vi "IR converter.vi"(1 "IR in":T1) -> (0 "distance out":T1)   [LabVIEW 2019]
uses:
  IR out.ctl
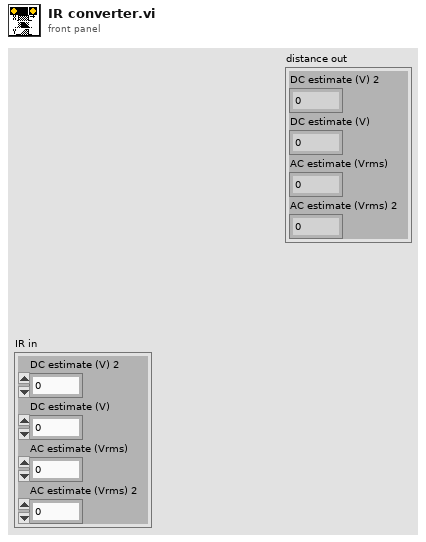
[diagram p1: front panel]
types:
  T1 = typedef "IR out.ctl" = cluster{"DC estimate (V) 2":dbl, "DC estimate (V)":dbl, "AC estimate (Vrms)":dbl, "AC estimate (Vrms) 2":dbl}
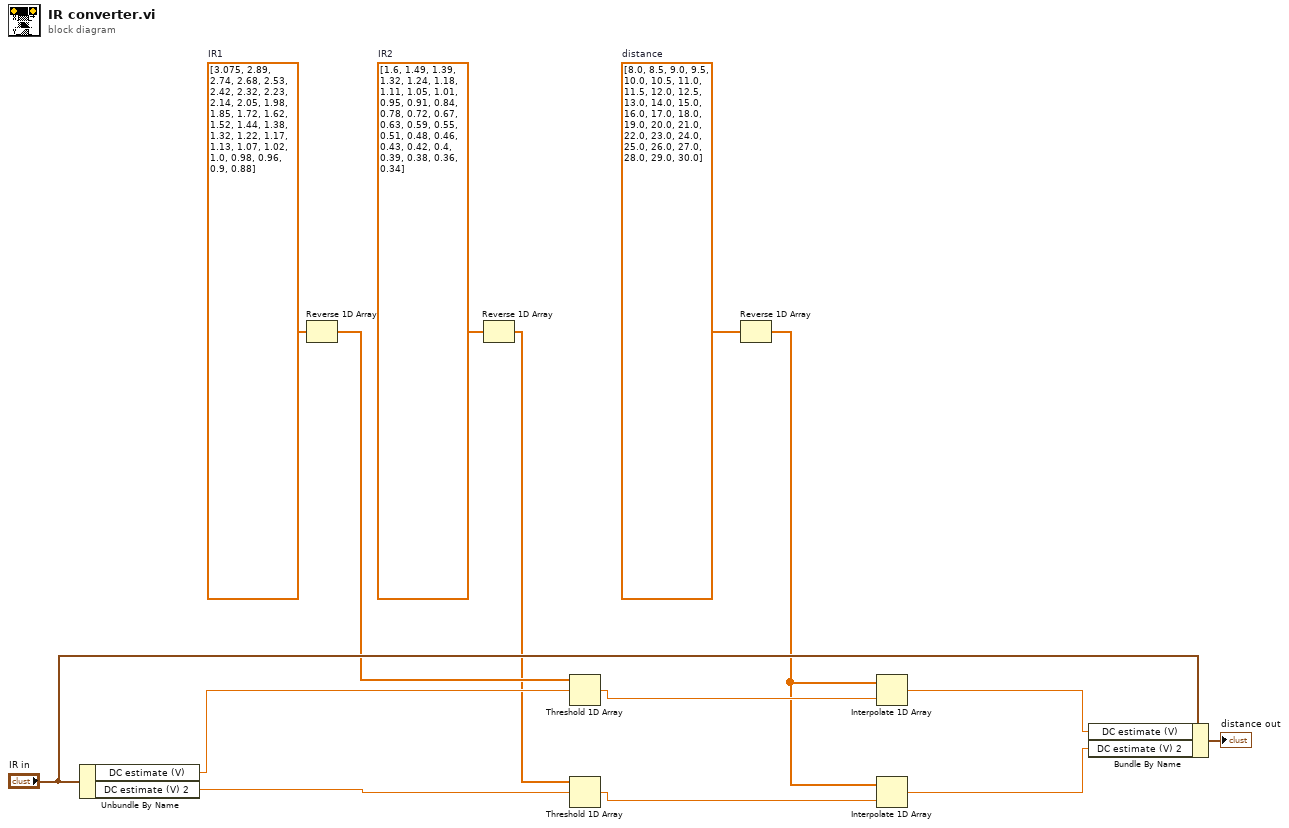
[diagram p0: block diagram]
diagram:
  w8 = dbl[] [1.6, 1.49, 1.39, 1.32, 1.24, 1.18, 1.11, 1.05, 1.01, 0.95, 0.91, 0.84, 0.78, 0.72, 0.67, 0.63, 0.59, 0.55, 0.51, 0.48, 0.46, 0.43, 0.42, 0.4, 0.39, 0.38, 0.36, 0.34]  # IR2
  w9 = dbl[] [3.075, 2.89, 2.74, 2.68, 2.53, 2.42, 2.32, 2.23, 2.14, 2.05, 1.98, 1.85, 1.72, 1.62, 1.52, 1.44, 1.38, 1.32, 1.22, 1.17, 1.13, 1.07, 1.02, 1.0, 0.98, 0.96, 0.9, 0.88]  # IR1
  w10 = dbl[] [8.0, 8.5, 9.0, 9.5, 10.0, 10.5, 11.0, 11.5, 12.0, 12.5, 13.0, 14.0, 15.0, 16.0, 17.0, 18.0, 19.0, 20.0, 21.0, 22.0, 23.0, 24.0, 25.0, 26.0, 27.0, 28.0, 29.0, 30.0]  # distance
  n1 = Unbundle By Name("IR in") -> ("DC estimate (V)"=w14:dbl, "DC estimate (V) 2"=w13:dbl)
  n2 = Reverse 1D Array(array=w9) -> (reversed array=w3:dbl[])
  n3 = Reverse 1D Array(array=w8) -> (reversed array=w2:dbl[])
  n4 = Threshold 1D Array(2:w14, 3:w3) -> (0:w11:dbl)  [unwired: 1 in]
  n5 = Threshold 1D Array(2:w13, 3:w2) -> (0:w12:dbl)  [unwired: 1 in]
  n6 = Reverse 1D Array(array=w10) -> (reversed array=w1:dbl[])
  n7 = Interpolate 1D Array(1:w11, 2:w1) -> (0:w6:dbl)
  n8 = Interpolate 1D Array(1:w12, 2:w1) -> (0:w5:dbl)
  n9 = Bundle By Name(cluster="IR in", "DC estimate (V)"=w6, "DC estimate (V) 2"=w5) -> (→"distance out":T1)
